vi "Remove Outliers (Range).vi"(0 "Y":dbl[](array[numeric]), 5 "X":dbl[](array[numeric]), 7 "Weight":dbl[](array[numeric]), 9 "range type":u16(ring) items=["Y", "X", "X and Y"], 11 "Range":dbl[](array[numeric])) -> (4 "Y Out":dbl[](array[numeric]), 6 "X Out":dbl[](array[numeric]), 8 "Weight Out":dbl[](array[numeric]), 10 "Outlier Indexes":i32[](array[numeric]), 15 "error":i32)   [LabVIEW 2017, in "NI_AALPro.lvlib"]
doc: "Removes data points that fall outside a given range or within a given index array. You must manually select the polymorphic instance you want to use."
uses:
  NI_AALPro.lvlib
  lvanlys.dll
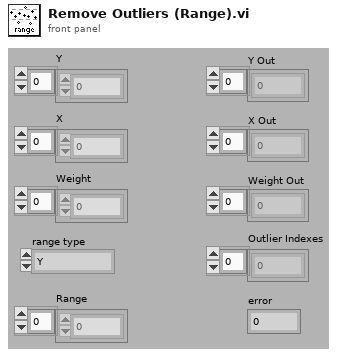
[diagram p1: front panel]
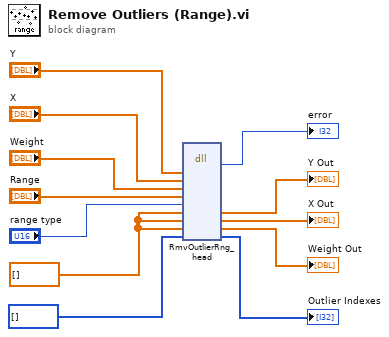
[diagram p0: block diagram]
diagram:
  w6 = dbl[] [] ("W Out")
  n1 = dll-call lib="C:/Program Files/National Instruments/LabVIEW 2017/resource/lvanlys.*" fn="RmvOutlierRng_head"("yIn"="Y", "xIn"="X", "wIn"="Weight", "range"="Range", "rangeType"="range type", "yOut"=w6, "xOut"=w6, "wOut"=w6, "outlierIndex"=i32[] [] ("Outliers")) -> (→"error":i32, "yOut"=→"Y Out":dbl[], "xOut"=→"X Out":dbl[], "wOut"=→"Weight Out":dbl[], "outlierIndex"=→"Outlier Indexes":i32[])  [unwired: 8 in, 2 out]
